vi "Set Aircraft Waypoints.vi"(8 "Error In":errorcluster, 10 "Waypoints In":T2(array[cluster]), 11 "Aircraft ID":u8) -> (0 "Error Out":errorcluster)   [LabVIEW 2014]
uses:
  MAVLink/Controls/MAVLINK Mav Frame.ctl
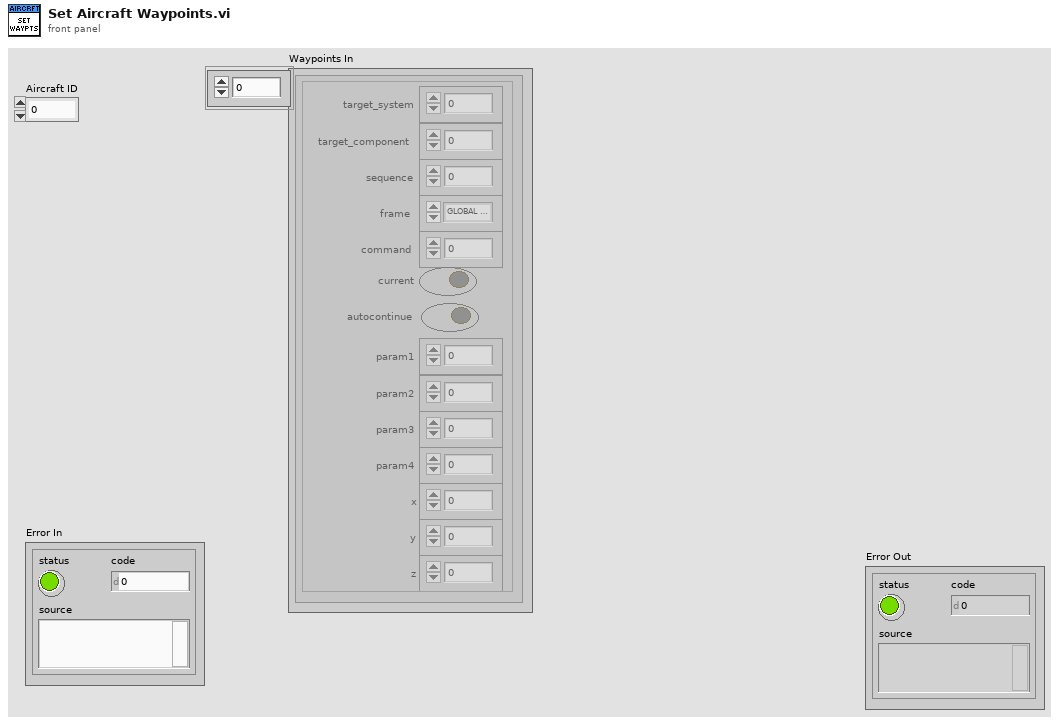
[diagram p1: front panel]
types:
  T1 = typedef "MAVLINK Mav Frame.ctl" = enum8{"GLOBAL", "LOCAL NED", "MISSION", "GLOBAL RELATIVE ALT", "LOCAL ENU", "GLOBAL INT", "GLOBAL RELATIVE ALT INT", "LOCAL OFFSET NED", "BODY NED", "BODY OFFSET NED", "GLOBAL TERRAIN ALT", "GLOBAL TERRAIN ALT INT"}
  T2 = cluster{"target_system":u8, "target_component":u8, "sequence":u16, "frame":T1, "command":u16, "current":bool, "autocontinue":bool, "param1":sgl, "param2":sgl, "param3":sgl, "param4":sgl, "x":sgl, "y":sgl, "z":sgl}[]
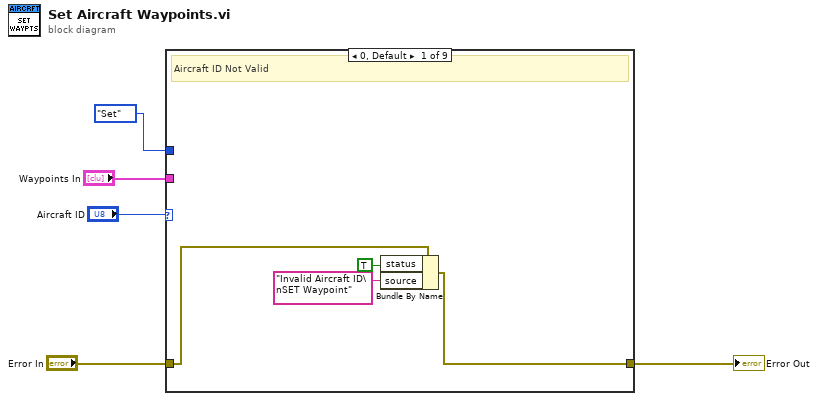
[diagram p0: block diagram]
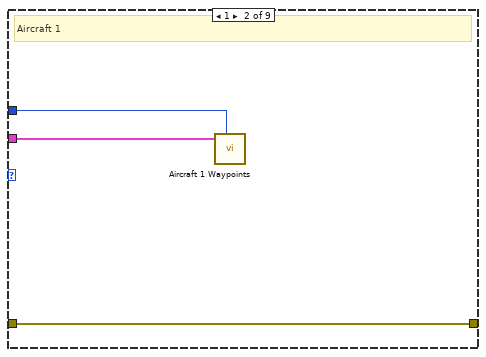
[diagram p2: hidden frame]
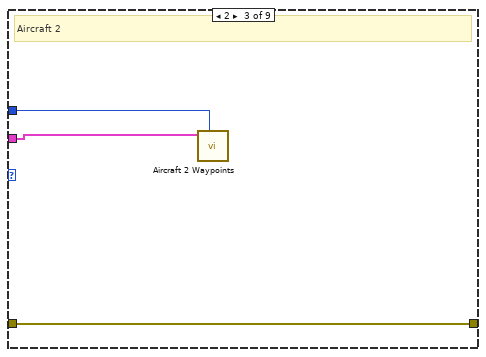
[diagram p3: hidden frame]
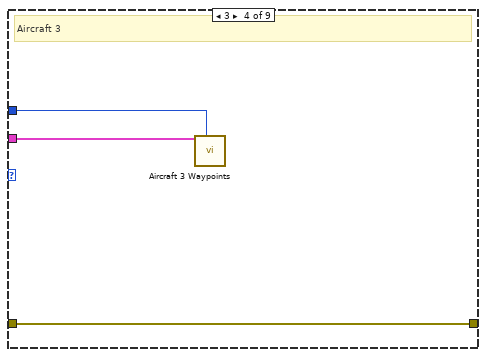
[diagram p4: hidden frame]
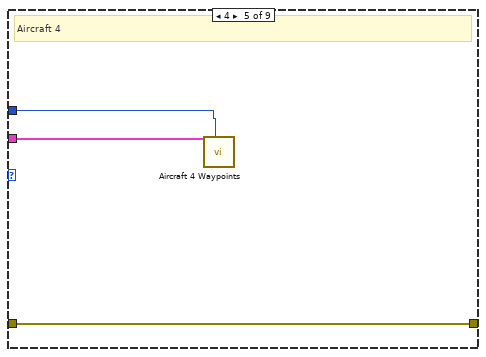
[diagram p5: hidden frame]
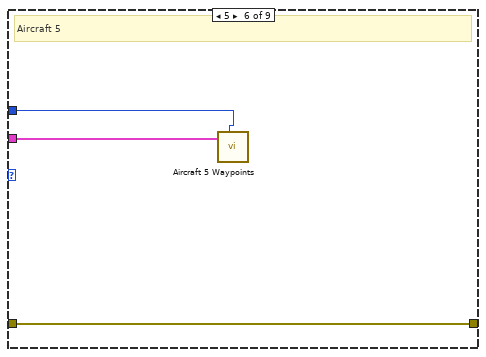
[diagram p6: hidden frame]
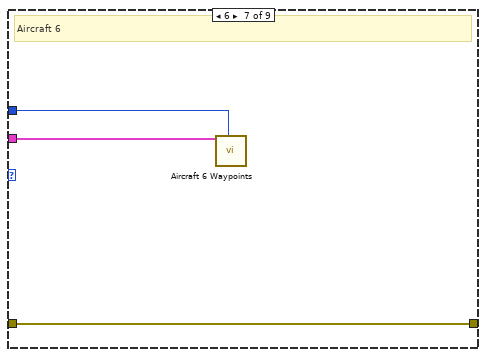
[diagram p7: hidden frame]
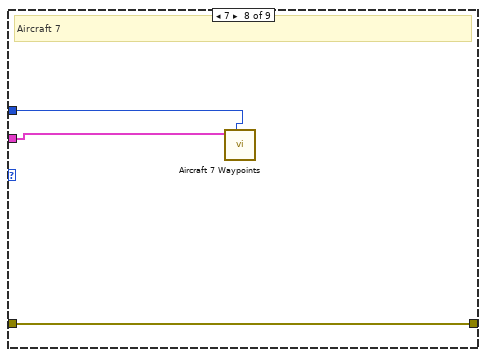
[diagram p8: hidden frame]
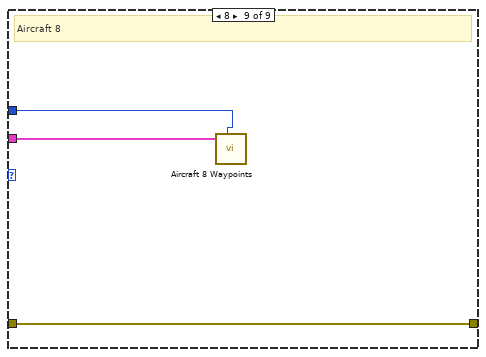
[diagram p9: hidden frame]
diagram:
  n1 = case shown="0, Default" "Aircraft ID" {
    tunnel: [w8 w12 w15 w18 w21 w24 w27 w30 w33] -> w4
    tunnel: "Error In" -> [w9 w12 w15 w18 w21 w24 w27 w30 w33]
    tunnel: enum16{"Get", "Set"}."Set" ("Method") -> [_ w11 w14 w17 w20 w23 w26 w29 w32]
    tunnel: "Waypoints In" -> [_ w10 w13 w16 w19 w22 w25 w28 w31]
    frame 0, Default {
      # "Aircraft ID Not Valid"
      n2 = Bundle By Name(cluster=w9, "status"=TRUE, "source"="Invalid Aircraft ID\nSET Waypoint") -> (w8:errorcluster)
    }
    frame 1 {
      # "Aircraft 1"
      n3 = call "Aircraft 1 Waypoints.vi"("Method"=w11, "Waypoints In"=w10) -> ()  [unwired: 9 in, 1 out]
    }
    frame 2 {
      # "Aircraft 2"
      n4 = call "Aircraft 2 Waypoints.vi"("Method"=w14, "Waypoints In"=w13) -> ()  [unwired: 9 in, 1 out]
    }
    frame 3 {
      # "Aircraft 3"
      n5 = call "Aircraft 3 Waypoints.vi"("Method"=w17, "Waypoints In"=w16) -> ()  [unwired: 9 in, 1 out]
    }
    frame 4 {
      # "Aircraft 4"
      n6 = call "Aircraft 4 Waypoints.vi"("Method"=w20, "Waypoints In"=w19) -> ()  [unwired: 9 in, 1 out]
    }
    frame 5 {
      # "Aircraft 5"
      n7 = call "Aircraft 5 Waypoints.vi"("Method"=w23, "Waypoints In"=w22) -> ()  [unwired: 9 in, 1 out]
    }
    frame 6 {
      # "Aircraft 6"
      n8 = call "Aircraft 6 Waypoints.vi"("Method"=w26, "Waypoints In"=w25) -> ()  [unwired: 9 in, 1 out]
    }
    frame 7 {
      # "Aircraft 7"
      n9 = call "Aircraft 7 Waypoints.vi"("Method"=w29, "Waypoints In"=w28) -> ()  [unwired: 9 in, 1 out]
    }
    frame 8 {
      # "Aircraft 8"
      n10 = call "Aircraft 8 Waypoints.vi"("Method"=w32, "Waypoints In"=w31) -> ()  [unwired: 9 in, 1 out]
    }
  }
  "Error Out" <- w4
